vi "ReportError Event Callback.vi"(4 "GUI.lvlib:Auto UI.lvlib:Auto UI.lvclass":refnum<class "Auto UI.lvclass">, 5 "Event data":cluster{"errorCode":i32, "errorMessage":string}, 6 "CtlRef":refnum<k7>, 7 "Event common data":cluster{"Source":i32, "Type":u32, "Time":u32}) -> ()   [LabVIEW 2023, in "GUI.lvlib" / "Auto UI.lvlib" / "Auto UI.lvclass"]
uses:
  Auto UI.lvclass
  Auto UI.lvclass/Auto UI.ctl
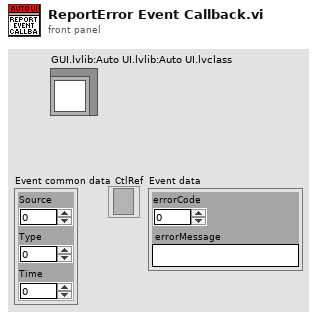
[diagram p1: front panel]
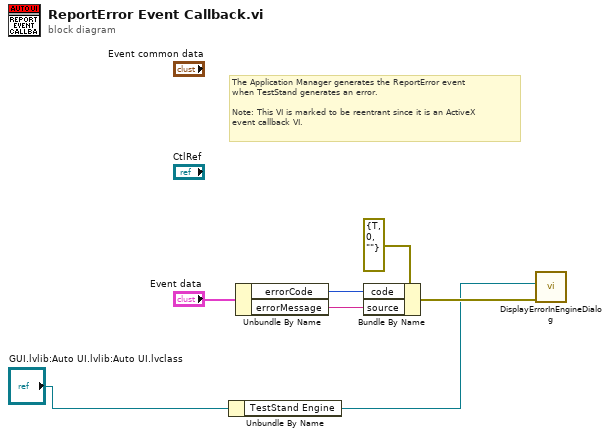
[diagram p0: block diagram]
diagram:
  # "The Application Manager generates the ReportError event\nwhen TestStand generates an error.\n\nNote: This VI is marked to be reentrant since it is an ActiveX\nevent callback VI."
  n1 = Unbundle By Name("GUI.lvlib:Auto UI.lvlib:Auto UI.lvclass") -> ("TestStand Engine"=w1:refnum<k7>)
  n2 = Unbundle By Name("Event data") -> ("errorCode"=w5:i32, "errorMessage"=w6:string)
  n3 = Bundle By Name(cluster=errorcluster {"status"=TRUE, "code"=0, "source"=""} ("error in (no error)"), "code"=w5, "source"=w6) -> (w2:errorcluster)
  n4 = call "DisplayErrorInEngineDialog.vi"("error in (no error)"=w2, "TestStand Engine"=w1) -> ()  [unwired: 10 in]
